vi "Read Traces.vi"(7 "max points":i32=1 min=1, 8 "error in (no error)":errorcluster, 9 "time interval":T1, 10 "PG path":string, 11 "Data.PGQL in":refnum<class "LV-Data.PGSQL.lvclass">) -> (0 "error out":errorcluster, 1 "Column (units)":string, 2 "Trace":cluster{timestamp[], dbl[]}[](array[cluster]), 3 "Data.PGSQL out":refnum<class "LV-Data.PGSQL.lvclass">, 5 "SQL string":string)   [LabVIEW 2019, in "LV-Data.PGSQL.lvclass"]
uses:
  LV-Data.PGSQL.lvclass
  Typedefs/Errors--enum.ctl
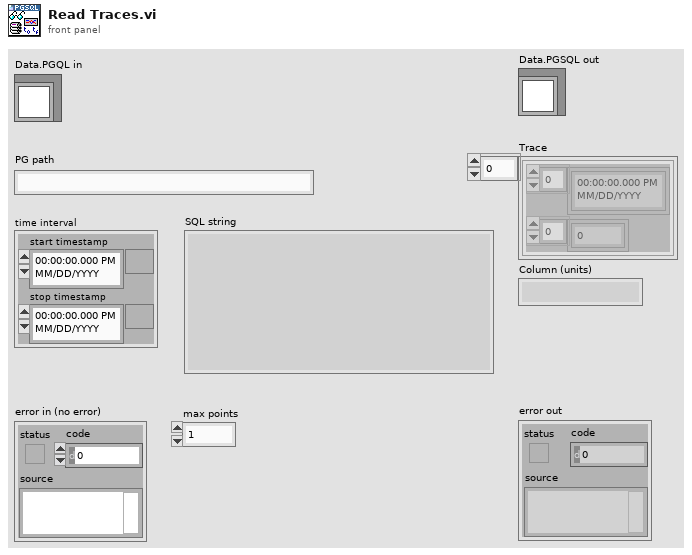
[diagram p1: front panel]
types:
  T1 = cluster{"start timestamp":timestamp, "stop timestamp":timestamp}
  T2 = typedef "LV-Data.PGSQL.lvclass/Time.Datatype--enum.ctl" = enum16{"timestamp without time zone", "timestamp with time zone"}
  T3 = typedef "LV-Data.PGSQL.lvclass/Errors--enum.ctl" = enum16{"0: None", "5005: Path Type Not Supported", "5006: Number of Variables", "5007: Number of data points", "5008: Cannot write two data points", "5030: Start and End Times Identical", "5031: Input is not wholly", "5032: Undefined Timestamps", "5033: Bad path or paths", "5040: Invalid Instrument Name", "5050: Column can only hold string", "5051: Column can only hold bool", "5052: Column can only hold double", "5053: Column can only hold int"}
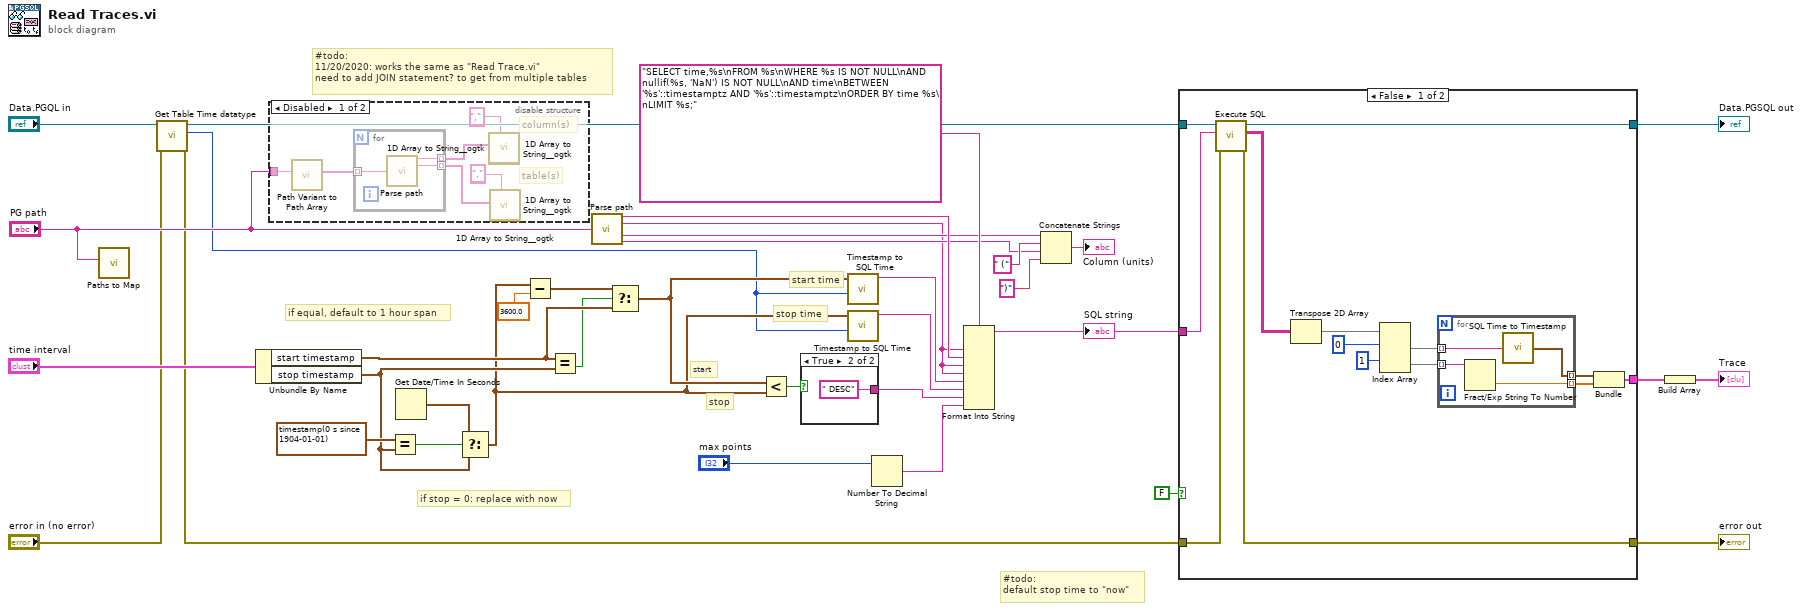
[diagram p0: block diagram]
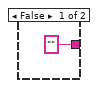
[diagram p3: hidden frame]
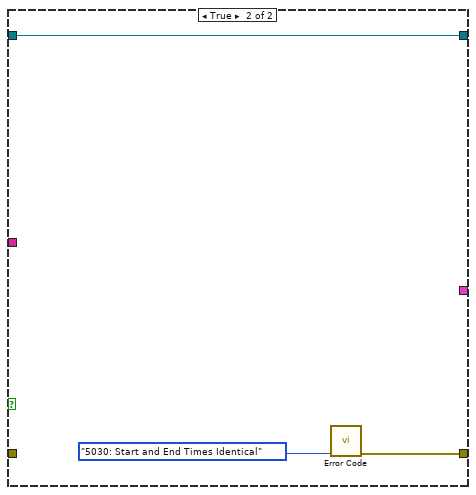
[diagram p4: hidden frame]
diagram:
  # "#todo:\n11/20/2020: works the same as \"Read Trace.vi\"\nneed to add JOIN statement? to get from multiple tables"
  # "if equal, default to 1 hour span"
  # "if stop = 0: replace with now"
  # "stop"
  # "start"
  # "stop time"
  # "start time"
  # "#todo:\ndefault stop time to \"now\""
  n1 = call "Paths to Map.vi"("Paths"="PG path") -> ()  [unwired: 9 in, 2 out]
  n2 = call "Get Table Time datatype.vi"("error in (no error)"="error in (no error)", "LV-Data.PGSQL in"="Data.PGQL in") -> ("error out"=w1:errorcluster, "Time Datatype"=w3:T2, "LV-Data.PGSQL out"=w4:refnum<class "LV-Data.PGSQL.lvclass">)  [unwired: 7 in]
  n3 = Unbundle By Name("time interval") -> ("start timestamp"=w14:timestamp, "stop timestamp"=w15:timestamp)
  n4 = disable-structure shown="Disabled" {
    disable-tunnel: "PG path" -> [w45 _]
    frame Disabled {
      # "table(s)"
      # "column(s)"
      n5 = call "Path Variant to Path Array.vi"("Paths"=w45) -> ("Paths"=w43:string[])  [unwired: 9 in, 1 out]
      n6 = for {
        tunnel: w43 -> [w48] mode=indexing
        tunnel: [w47] -> w42 mode=indexing
        tunnel: [w46] -> w38 mode=indexing
        n7 = call "Parse path.vi"("PG Path"=w48) -> ("Table path"=w47:string, "Column path"=w46:string)  [unwired: 10 in, 3 out]
      }
      n8 = call <userlib>:"1D Array to String__ogtk.vi"("delimiter (Tab)"=",", "Array of Strings"=w42) -> ()  [unwired: 9 in, 1 out]
      n9 = call <userlib>:"1D Array to String__ogtk.vi"("delimiter (Tab)"=",") -> ()  [unwired: 10 in, 1 out]
      n10 = call <userlib>:"1D Array to String__ogtk.vi"("delimiter (Tab)"=",") -> ()  [unwired: 10 in, 1 out]
      n11 = call <userlib>:"1D Array to String__ogtk.vi"("delimiter (Tab)"=",", "Array of Strings"=w38) -> ()  [unwired: 9 in, 1 out]
    }
    frame Enabled {
    }
  }
  n12 = Equal?(x=timestamp(0 s since 1904-01-01) ("stop timestamp"), y=w15) -> (x = y?=w20:bool)
  n13 = Get Date/Time In Seconds() -> (seconds since 1Jan1904=w17:timestamp)
  n14 = Select(t=w17, s=w20, f=w15) -> (s? t:f=w10:timestamp)
  n15 = Subtract(x=w10, y=3600.0) -> (x-y=w16:timestamp)
  n16 = Equal?(x=w14, y=w15) -> (x = y?=w13:bool)
  n17 = call "Parse path.vi"("PG Path"="PG path") -> ("Table path"=w30:string, "Column path"=w7:string, "Column name"=w28:string, "Column units"=w21:string)  [unwired: 10 in, 1 out]
  n18 = Select(t=w16, s=w13, f=w14) -> (s? t:f=w11:timestamp)
  n19 = Less?(x=w11, y=w10) -> (x < y?=w37:bool)
  n20 = case shown="True" w37 {
    tunnel: ["" " DESC"] -> w33
    frame False {
    }
    frame True {
    }
  }
  n21 = call "Timestamp to SQL Time.vi"("Time Datatype"=w3, "Timestamp"=w11) -> ("date/time string"=w24:string)  [unwired: 9 in]
  n22 = call "Timestamp to SQL Time.vi"("Time Datatype"=w3, "Timestamp"=w10) -> ("date/time string"=w23:string)  [unwired: 9 in]
  n23 = Number To Decimal String(number="max points") -> (decimal integer string=w34:string)  [unwired: 1 in]
  n24 = Format Into String(format string="SELECT time,%s\nFROM %s\nWHERE %s IS NOT NULL\nAND nullif(%s, 'NaN') IS NOT NULL\nAND time\nBETWEEN '%s'::timestamptz AND '%s'::timestamptz\nORDER BY time %s\nLIMIT %s;", w7, w30, w7, w7, w24, w23, w33, w34) -> (resulting string=w27:string)  [unwired: 2 in, 1 out]
  "SQL string" <- w27
  n25 = Concatenate Strings(w28, " (" ("string"), w21, ")" ("string")) -> (→"Column (units)":string)
  n26 = case shown="False" FALSE {
    tunnel: [w57 _] -> w36
    tunnel: w4 -> [w56 w71]
    tunnel: w27 -> [w52 _]
    tunnel: [w54 w69] -> w26
    tunnel: [w53 w71] -> w25
    tunnel: w1 -> [w55 _]
    frame False {
      n27 = call "Execute SQL.vi"("error in"=w55, "SQL"=w52, "LV-Data.PGSQL"=w56) -> ("error out"=w54:errorcluster, "Result"=w51:string[][], "LV-Data.PGSQL out"=w53:refnum<class "LV-Data.PGSQL.lvclass">)  [unwired: 6 in]
      n28 = Transpose 2D Array(2D array=w51) -> (transposed array=w64:string[][])
      n29 = Index Array(array=w64, index (row) #1=0 ("index (row)"), index (row) #2=1 ("index (row)")) -> (element #1=w61:string[], element #2=w60:string[])  [unwired: 2 in]
      n30 = for {
        tunnel: w61 -> [w68] mode=indexing
        tunnel: w60 -> [w67] mode=indexing
        tunnel: [w66] -> w58 mode=indexing
        tunnel: [w65] -> w59 mode=indexing
        n31 = Fract/Exp String To Number(string=w67) -> (number=w66:dbl)  [unwired: 3 in, 1 out]
        n32 = call "SQL Time to Timestamp.vi"("Get:Get String"=w68) -> ("Time Stamp"=w65:timestamp)
      }
      n33 = Bundle(w59, w58) -> (w57:cluster{timestamp[], dbl[]})  [unwired: 1 in]
    }
    frame True {
      n34 = call "Error Code.vi"("Error code"=Errors--enum."5030: Start and End Times Identical") -> ("error out"=w69:errorcluster)  [unwired: 10 in]
    }
  }
  "error out" <- w26
  "Data.PGSQL out" <- w25
  n35 = Build Array(w36) -> (→"Trace":cluster{timestamp[], dbl[]}[])
